vi "Main.vi"() -> ()   [LabVIEW 2015]
uses:
  <vilib>/Analysis/2dsp.llb/2D Complex FFT.vi
  <vilib>/Analysis/NI_AALPro.lvlib
panel:
  in  "Load memory":bool
  out "Trigger mode list":u32[](array[numeric])
  in  "Is record":bool
  in  "Trigger ON/OFF":bool
  in  "Trig send":bool
  in  "live stop":bool
  in  "live start":bool
  out "Error":bool
  out "satus":string
  out "reolsution":cluster{"Width":u32, "Height":u32}
  out "Error_Out":T1
  out "error out":errorcluster
  in  "Stop":bool
  in  "camera parameters":T2={"Setup"={"Shading:"=0, "Partition:"=1, "Shutter:"=0}, "camera"=0, "Head:"=0, "Resolution:"=4, "Frame Rate:"=0, "Camera Option"=FALSE} {"Frame Rate:" items=["50 fps", "60 fps", "125 fps", "250 fps", "500 fps", "1000 fps", "2000 fps", "3000 fps", "3600 fps", "4500 fps", "5000 fps", "6000 fps", "6750 fps", "8000 fps", "10000 fps", "13500 fps", "20000 fps", "30000 fps", "40000 fps", "50000 fps", "60000 fps", "75000 fps", "86400 fps", "100000 fps", "150000 fps", "225000 fps", "360000 fps", "500000 fps"]; "Resolution:" items=["1024 X 1024", "1024 X 896", "1024 X 800", "1024 X 640", "1024 X 512", "896 X 896", "896 X 752", "896 X 640", "896 X 512", "768 X 768", "768 X 640", "768 X 512", "640 X 640", "512 X 512", "512 X 384", "512 X 352", "384 X 288", "320 X 240", "320 X 192", "320 X 160", "320 X 128", "256 X 256", "256 X 128", "256 X 64", "192 X 128", "128 X 128", "128 X 96", "128 X 64", "128 X 32", "128 X 16", "64 X 16"]; "Head:" items=["Head No.0"]; "camera" items=["FASTCAM SA4 model 500K-M1"]; "Setup"."Shutter:" items=["1/50 sec", "1/60 sec", "1/100 sec", "1/200 sec", "1/300 sec", "1/400 sec", "1/500 sec", "1/600 sec", "1/700 sec", "1/800 sec", "1/900 sec", "1/1000 sec", "1/2000 sec", "1/3000 sec", "1/4000 sec", "1/5000 sec", "1/6000 sec", "1/7000 sec", "1/8000 sec", "1/9000 sec", "1/10000 sec", "1/12000 sec", "1/15000 sec", "1/17000 sec", "1/20000 sec", "1/25000 sec", "1/30000 sec", "1/34000 sec", "1/39000 sec", "1/50000 sec", "1/57000 sec", "1/62000 sec", "1/74000 sec", "1/82000 sec", "1/92000 sec", "1/104000 sec", "1/178000 sec", "1/333000 sec", "1/593000 sec", "1/1000000 sec"]; "Setup"."Shading:" items=["Shading"]; "Setup"."Partition:" items=["Partition 1"=1]}
  in  "Tab Control":enum32{"Page 1", "Page 2"}(tab)
  out "Intensity Graph 2":dbl[][](graph)
  out "Intensity Graph":u16[][](graph)
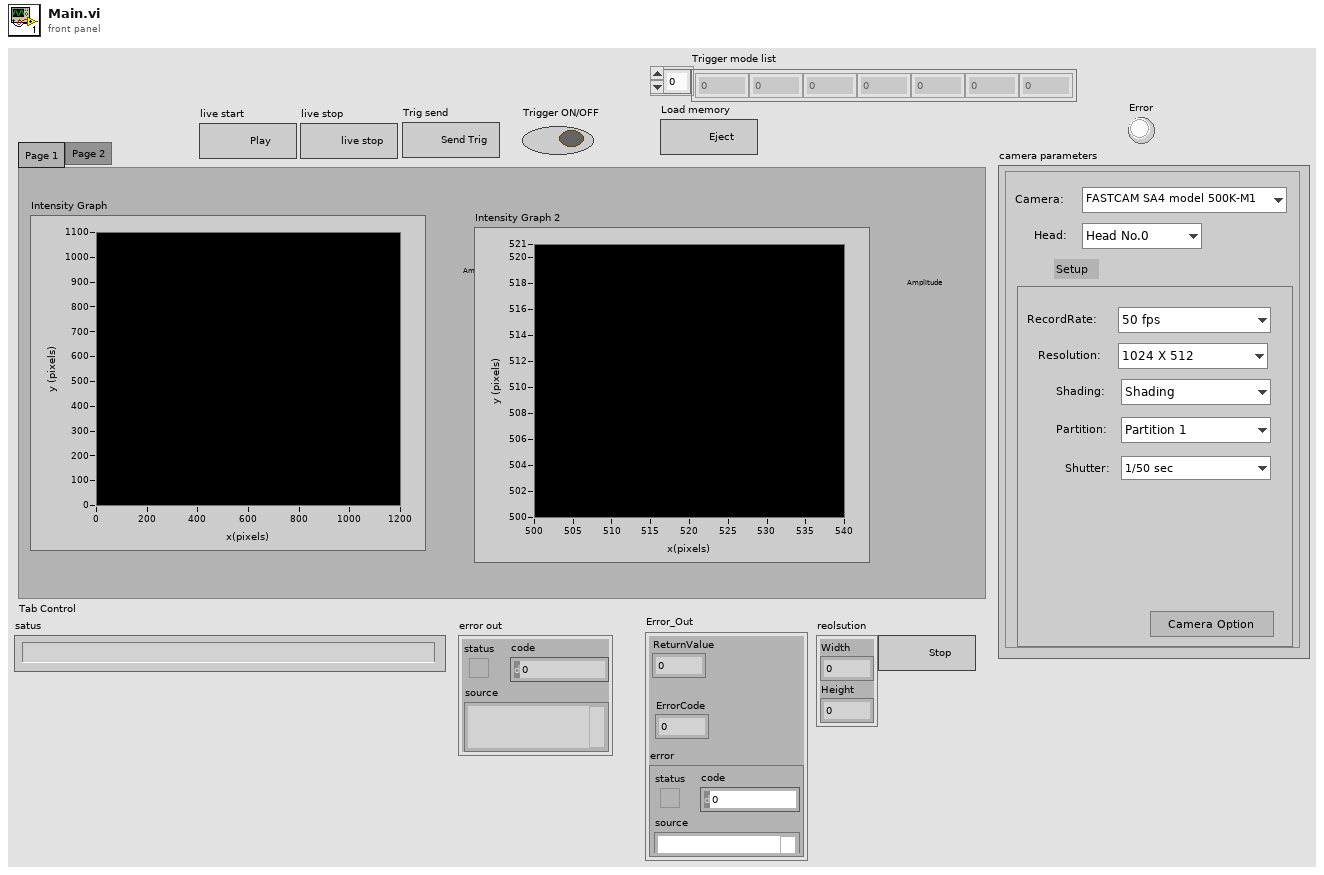
[diagram p1: front panel]
types:
  T1 = cluster{"ReturnValue":u32, "ErrorCode":u32, "error ":errorcluster}
  T2 = cluster{"Setup":cluster{"Shading:":u16, "Partition:":u16, "Shutter:":u16}, "camera":u16, "Head:":u16, "Resolution:":u16, "Frame Rate:":u16, "Camera Option":bool}
  T3 = cluster{"Detect Select BOX":enum32{"Detect Auto", "Detect Normal"}, "Auto_IP":cluster{"IP1":u8, "IP2":u8, "IP3":u8}, "Manual_IP":cluster{"IP1":u8, "IP2":u8, "IP3":u8, "IP4":u8}}
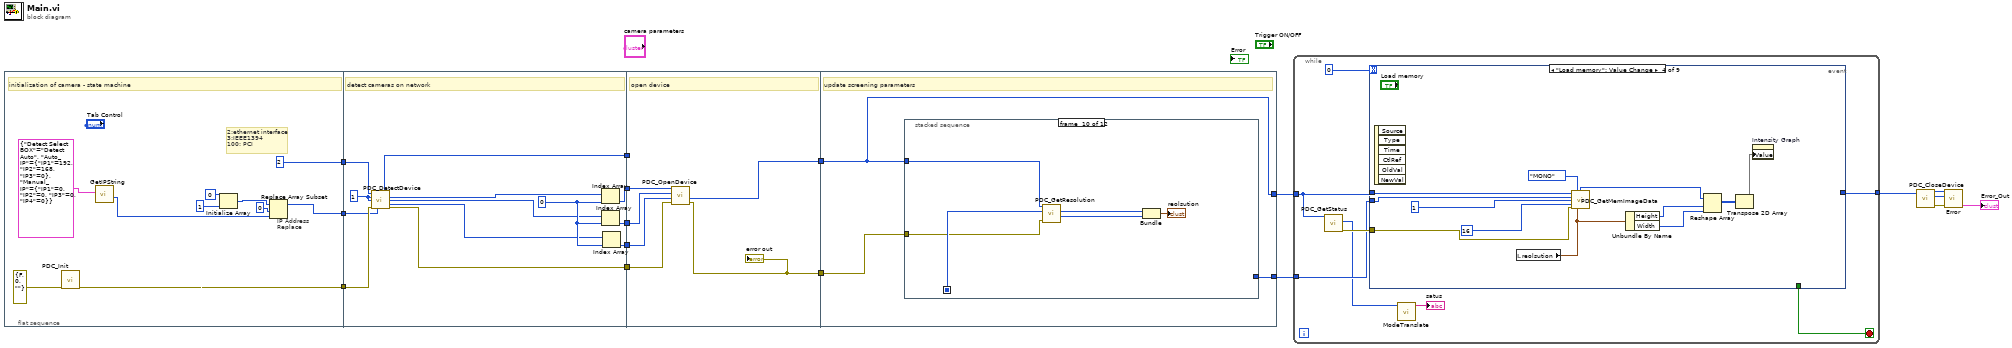
[diagram p0: block diagram]
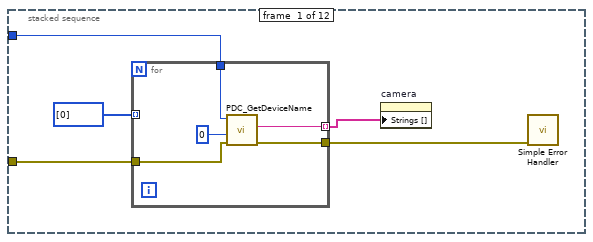
[diagram p2: hidden frame]
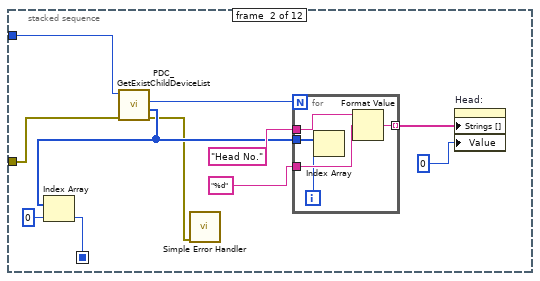
[diagram p3: hidden frame]
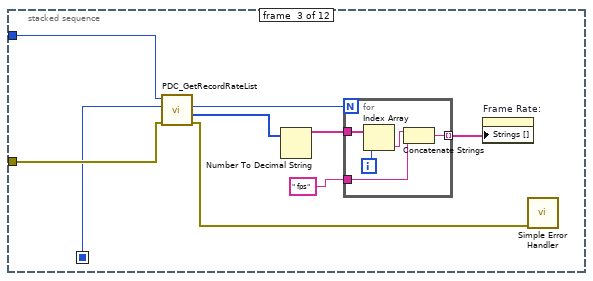
[diagram p4: hidden frame]
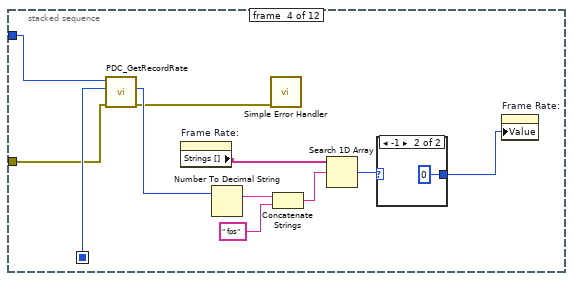
[diagram p5: hidden frame]
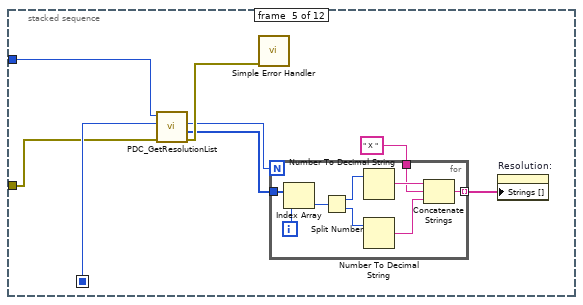
[diagram p7: hidden frame]
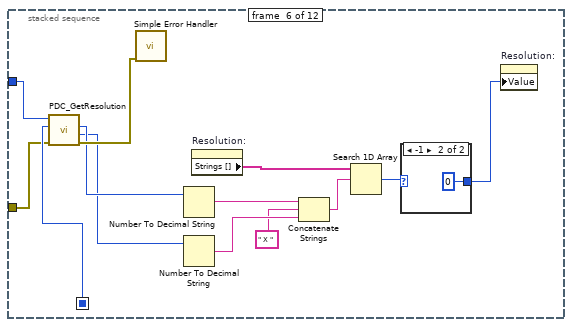
[diagram p8: hidden frame]
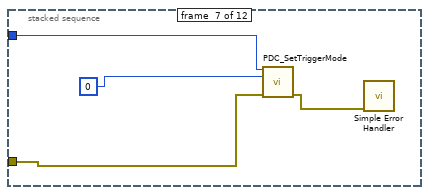
[diagram p10: hidden frame]
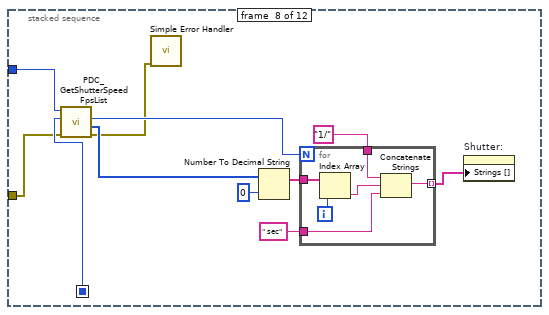
[diagram p11: hidden frame]
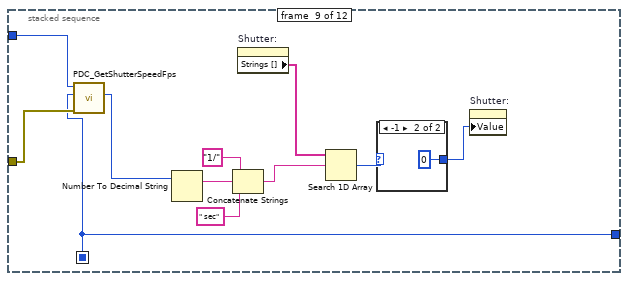
[diagram p12: hidden frame]
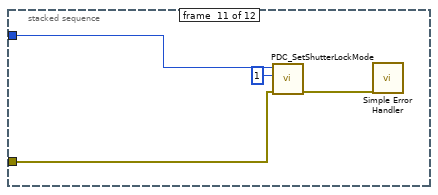
[diagram p14: hidden frame]
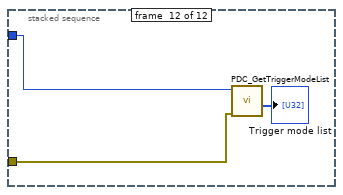
[diagram p15: hidden frame]
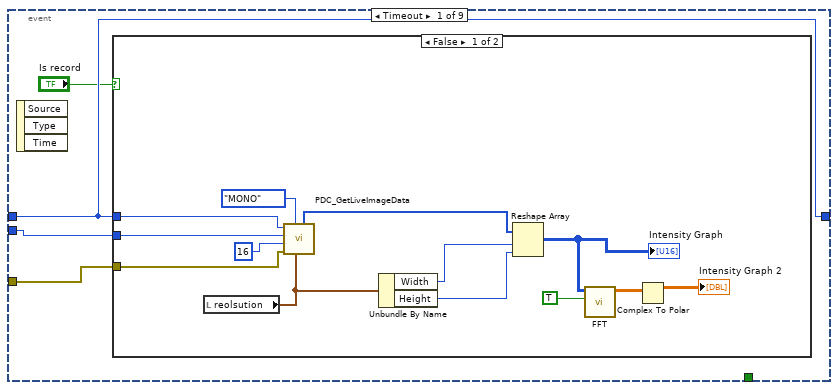
[diagram p16: hidden frame]
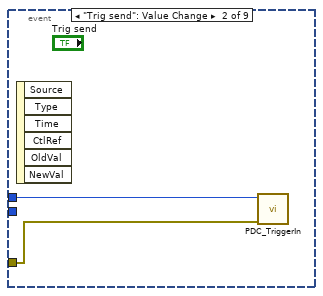
[diagram p18: hidden frame]
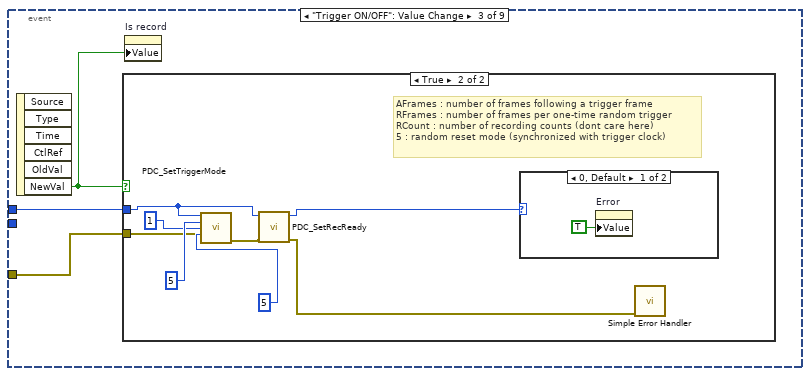
[diagram p19: hidden frame]
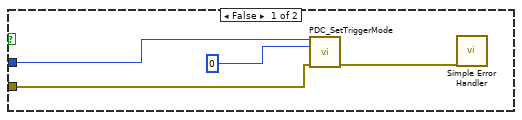
[diagram p20: hidden frame]
diagram:
  n1 = flat-sequence {
    tunnel: [u32 2 ("nInterfaceCode")] -> w17
    tunnel: [w18] -> w16
    tunnel: [w22] -> w15
    tunnel: w17 -> [w38]
    tunnel: w16 -> [w40]
    tunnel: w15 -> [w36]
    tunnel: [w37] -> w14
    tunnel: [w35] -> w13
    tunnel: [w34] -> w12
    tunnel: [w32] -> w11
    tunnel: [w31] -> w2
    tunnel: w14 -> [w43]
    tunnel: w13 -> [w46]
    tunnel: w12 -> [w45]
    tunnel: w11 -> [w44]
    tunnel: [w42] -> w4
    tunnel: [w41] -> w3
    tunnel: w2 -> [_]
    tunnel: [w49] -> w6
    tunnel: w4 -> [w49]
    tunnel: w3 -> [w48]
    tunnel: [w47] -> w1
    frame #0 {
      # "2:ethernet interface\n3:IEEE1394\n100: PCI"
      # "IP Address\nReplace"
      # "initialization of camera - state machine"
      n2 = call "PDC_Init.vi"("error in (no error)"=errorcluster {"status"=FALSE, "code"=0, "source"=""}) -> ("error out"=w18:errorcluster)  [unwired: 10 out]
      n3 = call "GetIPString.vi"("Out_IP Address"=T3 {"Detect Select BOX"=enum."Detect Auto", "Auto_IP"={"IP1"=192, "IP2"=168, "IP3"=0}, "Manual_IP"={"IP1"=0, "IP2"=0, "IP3"=0, "IP4"=0}}) -> ("Net address"=w27:u32)  [unwired: 10 out]
      n4 = Initialize Array "Initialize Array"(u32 0 ("要素"), 1 ("dimension size")) -> (w25:u32[])
      n5 = Replace Array Subset "Replace Array Subset"(array=w25, new element=w27, index=0 ("指標")) -> (w22:u32[])
    }
    frame #1 {
      w33 = 0 ("index")
      w39 = u32 1 ("DetectNum")
      # "detect cameras on network"
      n6 = call "PDC_DetectDevice.vi"("InterfaceCode"=w38, "DetectNum"=w39, "DetectParam"=w39, "error in (no error)"=w40, "DetectNo"=w36) -> ("DeviceNum"=w31:u32, "DeviceCode"=w28:u32[], "TmpDeviceNo"=w30:u32[], "InterfaceCode(out)"=w29:u32[], "error out"=w37:errorcluster)  [unwired: 4 in, 2 out]
      n7 = Index Array(array=w28, index=w33) -> (element=w35:u32)
      n8 = Index Array(array=w30, index=w33) -> (element=w34:u32)
      n9 = Index Array(array=w29, index=w33) -> (element=w32:u32)
    }
    frame #2 {
      # "open device"
      n10 = call "PDC_OpenDevice.vi"("error in (no error)"=w43, "InterfaceCode"=w44, "TmpDeviceNo"=w45, "DeviceCode"=w46) -> ("error out"=w41:errorcluster, "DeviceNo"=w42:u32)  [unwired: 6 out]
      "error out" <- w41
    }
    frame #3 {
      # "update screening parameters"
      n11 = stacked-sequence {
        seq-local: [_ w61 _ _ _ _ _ _ _ _ _ _] -> [_ _ w77 w99 w107 w131 _ w148 w156 w173 _ _]
        tunnel: w49 -> [w54 w70 w84 w100 w108 w132 w138 w149 w166 w174 w178 w181]
        tunnel: w48 -> [w53 w69 w83 w98 w106 w130 w137 w147 w165 w172 w176 w180]
        tunnel: [_ _ _ _ _ _ _ _ w156 _ _ _] -> w47
        frame #0 {
          n12 = for {
            tunnel: w54 -> [w59]
            tunnel: w53 -> [w58]
            tunnel: [w56] -> w51 mode=indexing
            tunnel: u32[] [0] ("nDeviceNoList 2") -> [_] mode=indexing
            tunnel: [w55] -> w50
            n13 = call "PDC_GetDeviceName.vi"("error in (no error)"=w58, "ChildNo"=u32 0, "DeviceNo"=w59) -> ("error out"=w55:errorcluster, "StrName"=w56:string)  [unwired: 1 in, 6 out]
          }
          n14 = property on="camera" class="Ring (strict)"("Strings []"=w51) -> ()  [unwired: 2 in, 2 out]
          n15 = call <vilib>:"Simple Error Handler.vi"("error in (no error)"=w50) -> ()  [unwired: 4 in, 5 out]
        }
        frame #1 {
          n16 = call "PDC_GetExistChildDeviceList.vi"("error in (no error)"=w69, "DeviceNo"=w70) -> ("error out"=w60:errorcluster, "List"=w63:u32[], "Size"=w66:u32)  [unwired: 7 out]
          n17 = Index Array(array=w63, index=0) -> (element=w61:u32)
          n18 = call <vilib>:"Simple Error Handler.vi"("error in (no error)"=w60) -> ()  [unwired: 4 in, 5 out]
          n19 = for {
            N: w66 -> [_]
            tunnel: "Head No." -> [w75]
            tunnel: "%d" -> [w74]
            tunnel: [w73] -> w65 mode=indexing
            tunnel: w63 -> [w71]
            i -> [w72]
            n20 = Index Array(array=w71, index=w72) -> ()  [unwired: 1 out]
            n21 = Format Value(string ("")=w75, format string=w74) -> (output string=w73:string)  [unwired: 1 in]
          }
          n22 = property on="Head:" class="Ring (strict)"("Strings []"=w65, "Value"=u32 0 ("値")) -> ()  [unwired: 2 in, 2 out]
        }
        frame #2 {
          n23 = call "PDC_GetRecordRateList.vi"("error in (no error)"=w83, "ChildNo"=w77, "DeviceNo"=w84) -> ("error out"=w76:errorcluster, "List"=w79:u32[], "Size"=w80:u32)  [unwired: 6 out]
          n24 = Number To Decimal String(number=w79) -> (decimal integer string=w82:string[])  [unwired: 1 out]
          n25 = for {
            N: w80 -> [_]
            tunnel: w82 -> [w86]
            tunnel: [w89] -> w78 mode=indexing
            tunnel: " fps" -> [w88]
            i -> [w87]
            n26 = Index Array(array=w86, index=w87) -> (element=w85:string)
            n27 = Concatenate Strings(w85, w88) -> (w89:string)
          }
          n28 = property on="Frame Rate:" class="Ring (strict)"("Strings []"=w78) -> ()  [unwired: 2 in, 2 out]
          n29 = call <vilib>:"Simple Error Handler.vi"("error in (no error)"=w76) -> ()  [unwired: 4 in, 5 out]
        }
        frame #3 {
          n30 = call "PDC_GetRecordRate.vi"("error in (no error)"=w98, "ChildNo"=w99, "DeviceNo"=w100) -> ("error out"=w90:errorcluster, "Rate"=w91:u32)  [unwired: 7 out]
          n31 = property on="Frame Rate:" class="Ring (strict)"() -> ("Strings []"=w93:string[])  [unwired: 2 in, 2 out]
          n32 = Number To Decimal String(number=w91) -> (decimal integer string=w96:string)  [unwired: 1 out]
          n33 = call <vilib>:"Simple Error Handler.vi"("error in (no error)"=w90) -> ()  [unwired: 4 in, 5 out]
          n34 = Concatenate Strings(w96, " fps") -> (w95:string)
          n35 = Search 1D Array(1D array=w93, element=w95) -> (index of element=w94:i32)  [unwired: 1 out]
          n36 = case shown="-1" w94 {
            selector: w94 -> [w101 _]
            tunnel: [w101 0 ("index of element")] -> w92
            frame Default {
            }
            frame -1 {
            }
          }
          n37 = property on="Frame Rate:" class="Ring (strict)"("Value"=w92) -> ()  [unwired: 2 in, 2 out]
        }
        frame #4 {
          n38 = call "PDC_GetResolutionList.vi"("error in (no error)"=w106, "ChildNo"=w107, "DeviceNo"=w108) -> ("error out"=w105:errorcluster, "List"=w103:u32[], "Size"=w104:u32)  [unwired: 6 out]
          n39 = call <vilib>:"Simple Error Handler.vi"("error in (no error)"=w105) -> ()  [unwired: 4 in, 5 out]
          n40 = for {
            N: w104 -> [_]
            tunnel: " X " -> [w117]
            tunnel: [w116] -> w109 mode=indexing
            tunnel: w103 -> [w112]
            i -> [w115]
            n41 = Index Array(array=w112, index=w115) -> (element=w111:u32)
            n42 = Split Number(x=w111) -> (hi(x)=w114:u16, lo(x)=w113:u16)
            n43 = Number To Decimal String(number=w114) -> (decimal integer string=w119:string)  [unwired: 1 out]
            n44 = Number To Decimal String(number=w113) -> (decimal integer string=w118:string)  [unwired: 1 out]
            n45 = Concatenate Strings(w119, w117, w118) -> (w116:string)
          }
          n46 = property on="Resolution:" class="Ring (strict)"("Strings []"=w109) -> ()  [unwired: 2 in, 2 out]
        }
        frame #5 {
          n47 = call "PDC_GetResolution.vi"("error in (no error)"=w130, "ChildNo"=w131, "DeviceNo"=w132) -> ("error out"=w129:errorcluster, "Height"=w122:u32, "Width"=w123:u32)  [unwired: 6 out]
          n48 = call <vilib>:"Simple Error Handler.vi"("error in (no error)"=w129) -> ()  [unwired: 4 in, 5 out]
          n49 = Number To Decimal String(number=w123) -> (decimal integer string=w126:string)  [unwired: 1 out]
          n50 = Number To Decimal String(number=w122) -> (decimal integer string=w127:string)  [unwired: 1 out]
          n51 = property on="Resolution:" class="Ring (strict)"() -> ("Strings []"=w121:string[])  [unwired: 2 in, 2 out]
          n52 = Concatenate Strings(w126, " X ", w127) -> (w124:string)
          n53 = Search 1D Array(1D array=w121, element=w124) -> (index of element=w128:i32)  [unwired: 1 in]
          n54 = case shown="-1" w128 {
            selector: w128 -> [w133 _]
            tunnel: [w133 0 ("index of element")] -> w120
            frame Default {
            }
            frame -1 {
            }
          }
          n55 = property on="Resolution:" class="Ring (strict)"("Value"=w120) -> ()  [unwired: 2 in, 2 out]
        }
        frame #6 {
          n56 = call "PDC_SetTriggerMode.vi"("DeviceNo"=w138, "Mode"=u32 0 ("nMode"), "error in (no error)"=w137) -> ("error out"=w135:errorcluster)  [unwired: 3 in, 9 out]
          n57 = call <vilib>:"Simple Error Handler.vi"("error in (no error)"=w135) -> ()  [unwired: 4 in, 5 out]
        }
        frame #7 {
          n58 = call "PDC_GetShutterSpeedFpsList.vi"("error in (no error)"=w147, "ChildNo"=w148, "DeviceNo"=w149) -> ("error out"=w139:errorcluster, "List"=w142:u32[], "Size"=w141:u32)  [unwired: 6 out]
          n59 = call <vilib>:"Simple Error Handler.vi"("error in (no error)"=w139) -> ()  [unwired: 4 in, 5 out]
          n60 = Number To Decimal String(number=w142, width (-)=u32 0 ("幅（-）")) -> (decimal integer string=w146:string[])
          n61 = for {
            N: w141 -> [_]
            tunnel: w146 -> [w151]
            tunnel: [w155] -> w140 mode=indexing
            tunnel: "1/" -> [w153]
            tunnel: " sec" -> [w152]
            i -> [w154]
            n62 = Index Array(array=w151, index=w154) -> (element=w150:string)
            n63 = Concatenate Strings(w153, w150, w152) -> (w155:string)
          }
          n64 = property on="Shutter:" class="Ring (strict)"("Strings []"=w140) -> ()  [unwired: 2 in, 2 out]
        }
        frame #8 {
          n65 = call "PDC_GetShutterSpeedFps.vi"("error in (no error)"=w165, "ChildNo"=w156, "DeviceNo"=w166) -> ("Fps"=w157:u32)  [unwired: 8 out]
          n66 = Number To Decimal String(number=w157) -> (decimal integer string=w160:string)  [unwired: 1 out]
          n67 = Concatenate Strings("1/", w160, " sec") -> (w163:string)
          n68 = property on="Shutter:" class="Ring (strict)"() -> ("Strings []"=w158:string[])  [unwired: 2 in, 2 out]
          n69 = Search 1D Array(1D array=w158, element=w163) -> (index of element=w162:i32)  [unwired: 1 out]
          n70 = case shown="-1" w162 {
            selector: w162 -> [w167 _]
            tunnel: [w167 0 ("index of element")] -> w159
            frame Default {
            }
            frame -1 {
            }
          }
          n71 = property on="Shutter:" class="Ring (strict)"("Value"=w159) -> ()  [unwired: 2 in, 2 out]
        }
        frame #9 {
          n72 = call "PDC_GetResolution.vi"("error in (no error)"=w172, "ChildNo"=w173, "DeviceNo"=w174) -> ("Height"=w170:u32, "Width"=w171:u32)  [unwired: 7 out]
          n73 = Bundle("Width"=w171, "Height"=w170) -> (→"reolsution":cluster{"Width":u32, "Height":u32})  [unwired: 1 in]
        }
        frame #10 {
          n74 = call "PDC_SetShutterLockMode.vi"("error in (no error)"=w176, "Mode"=u32 1, "DeviceNo"=w178) -> ("error out"=w175:errorcluster)  [unwired: 6 in, 2 out]
          n75 = call <vilib>:"Simple Error Handler.vi"("error in (no error)"=w175) -> ()  [unwired: 4 in, 5 out]
        }
        frame #11 {
          n76 = call "PDC_GetTriggerModeList.vi"("error in (no error)"=w180, "DeviceNo"=w181) -> ("List"=→"Trigger mode list":u32[])  [unwired: 5 in, 4 out]
        }
      }
    }
  }
  n77 = while {
    tunnel: [w187] -> w7
    tunnel: w6 -> [w188]
    tunnel: w1 -> [w184]
    stop <- w185 stop-if-true
    n78 = call "PDC_GetStatus.vi"("DeviceNo"=w188) -> ("error out"=w186:errorcluster, "Status"=w183:u32)  [unwired: 1 in, 8 out]
    n79 = event shown="[3] \"Load memory\": Value Change" {
      selector: _ -> [_ _ _ _ _ _ _ _ _]
      dyn-events: _ -> [_ _ _ _ _ _ _ _ _]
      timeout: 0 -> [_ _ _ _ _ _ _ _ _]
      tunnel: w188 -> [w192 w208 w211 w236 w241 w244 w247 w268 w269]
      tunnel: [w192 _ _ _ _ _ w247 _ w269] -> w187
      tunnel: w186 -> [w193 w207 w210 w231 w240 w243 w255 w266 _]
      tunnel: [_ _ _ _ _ _ _ _ TRUE] -> w185
      tunnel: w184 -> [w191 _ _ w234 _ _ w246 w267 _]
      event Timeout {
        n80 = event-data() -> ()  [unwired: 1 in, 3 out]
        n81 = case shown="False" "Is record" {
          tunnel: w193 -> [w204 _]
          tunnel: w192 -> [w199 _]
          tunnel: w191 -> [w198 _]
          frame False {
            n82 = local read "reolsution"() -> (w202:cluster{"Width":u32, "Height":u32})
            n83 = call "PDC_GetLiveImageData.vi"("Resolution"=w202, "ColorType"=enum16{"MONO", "COLOR"}."MONO", "error in (no error)"=w204, "BitDepth"=u32 16, "ChildNo"=w198, "DeviceNo"=w199) -> ("Data(16Bit)"=w203:u16[])  [unwired: 5 out]
            n84 = Unbundle By Name(w202) -> ("Width"=w201:u32, "Height"=w200:u32)
            n85 = Reshape Array(w203, w201, w200) -> (w197:u16[][])
            "Intensity Graph" <- w197
            n86 = call-poly <vilib>:"FFT.vi"("shift?"=TRUE, "X"=w197) -> ("FFT {X}"=w196:cdb[][])  [unwired: 8 in, 1 out]
            n87 = Complex To Polar(r * e^(i*theta)=w196) -> (r=→"Intensity Graph 2":dbl[][])  [unwired: 1 out]
          }
          frame True {
          }
        }
      }
      event "Trig send": Value Change {
        n88 = event-data() -> ()  [unwired: 1 in, 6 out]
        n89 = call "PDC_TriggerIn.vi"("error in (no error)"=w207, "DeviceNo"=w208) -> ()  [unwired: 7 in, 3 out]
      }
      event "Trigger ON/OFF": Value Change {
        n90 = event-data() -> ("NewVal"=w209:bool)  [unwired: 1 in, 5 out]
        n91 = case shown="True" w209 {
          tunnel: w211 -> [w214 w216]
          tunnel: w210 -> [w212 w220]
          frame False {
            n92 = call "PDC_SetTriggerMode.vi"("DeviceNo"=w214, "Mode"=u32 0, "error in (no error)"=w212) -> ("error out"=w215:errorcluster)  [unwired: 10 in, 2 out]
            n93 = call <vilib>:"Simple Error Handler.vi"("error in (no error)"=w215) -> ()  [unwired: 4 in, 5 out]
          }
          frame True {
            # "AFrames : number of frames following a trigger frame\nRFrames : number of frames per one-time random trigger\nRCount : number of recording counts (dont care here)\n5 : random reset mode (synchronized with trigger clock)"
            n94 = call "PDC_SetTriggerMode.vi"("DeviceNo"=w216, "Mode"=u32 5, "AFrames"=u32 1, "RFrames"=u32 5, "error in (no error)"=w220) -> ("error out"=w219:errorcluster)  [unwired: 8 in, 2 out]
            n95 = call "PDC_SetRecReady.vi"("error in (no error)"=w219, "DeviceNo"=w216) -> ("error out"=w218:errorcluster, "ReturnValue"=w217:u32)  [unwired: 7 in, 1 out]
            n96 = case shown="0, Default" w217 {
              frame 0, Default {
                n97 = property on="Error" class="Bool (strict)"("Value"=TRUE ("Error")) -> ()  [unwired: 2 in, 2 out]
              }
              frame 1 {
              }
            }
            n98 = call <vilib>:"Simple Error Handler.vi"("error in (no error)"=w218) -> ()  [unwired: 4 in, 5 out]
          }
        }
        n99 = property on="Is record" class="Bool (strict)"("Value"=w209) -> ()  [unwired: 2 in, 2 out]
      }
      event "Load memory": Value Change {
        n100 = event-data() -> ()  [unwired: 1 in, 6 out]
        n101 = local read "reolsution"() -> (w230:cluster{"Width":u32, "Height":u32})
        n102 = call "PDC_GetMemImageData.vi"("DeviceNo"=w236, "ColorType"=enum16{"MONO", "COLOR"}."MONO", "ChildNo"=w234, "FrameNo"=1, "BitDepth"=u32 16, "error in (no error)"=w231, "Resolution"=w230) -> ("Data(16Bit)"=w227:u16[])  [unwired: 4 in, 4 out]
        n103 = Unbundle By Name(w230) -> ("Height"=w229:u32, "Width"=w228:u32)
        n104 = Reshape Array(w227, w229, w228) -> (w226:u16[][])
        n105 = Transpose 2D Array(2D array=w226) -> (transposed array=w225:u16[][])
        n106 = property on="Intensity Graph" class="IntGraph (strict)"("Value"=w225) -> ()  [unwired: 2 in, 2 out]
      }
      event "live stop": Value Change {
        n107 = event-data() -> ()  [unwired: 1 in, 6 out]
        n108 = call "PDC_SetStatus.vi"("error in (no error)"=w240, "Mode"=u32 1, "DeviceNo"=w241) -> ("error out"=w239:errorcluster)  [unwired: 8 out]
        n109 = call <vilib>:"Simple Error Handler.vi"("error in (no error)"=w239) -> ()  [unwired: 4 in, 5 out]
        n110 = property on="Is record" class="Bool (strict)"("Value"=TRUE ("Is live")) -> ()  [unwired: 2 in, 2 out]
      }
      event "live start": Value Change {
        n111 = event-data() -> ()  [unwired: 1 in, 6 out]
        n112 = call "PDC_SetStatus.vi"("error in (no error)"=w243, "Mode"=u32 0, "DeviceNo"=w244) -> ()  [unwired: 9 out]
        n113 = property on="Is record" class="Bool (strict)"("Value"=FALSE ("Is live")) -> ()  [unwired: 2 in, 2 out]
      }
      event "camera parameters.Frame Rate:": Value Change {
        n114 = event-data() -> ()  [unwired: 1 in, 6 out]
        n115 = property on="Frame Rate:" class="Ring (strict)"() -> ("Strings []"=w250:string[], "Value"=w249:u16)  [unwired: 2 in, 2 out]
        n116 = Index Array(array=w250, index=w249) -> (element=w254:string)
        n117 = Match Pattern(string=w254, regular expression=" fps") -> (before substring=w252:string)  [unwired: 4 out]
        n118 = Decimal String To Number(string=w252, default (0L)=u32 0 ("デフォルト (0 I32)")) -> (number=w248:u32)  [unwired: 2 out]
        n119 = call "PDC_SetRecordRate.vi"("error in (no error)"=w255, "Rate"=w248, "ChildNo"=w246, "DeviceNo"=w247) -> ("error out"=w256:errorcluster)  [unwired: 7 out]
        n120 = call <vilib>:"Simple Error Handler.vi"("error in (no error)"=w256) -> ()  [unwired: 4 in, 5 out]
      }
      event "camera parameters.Setup.Shutter:": Value Change {
        n121 = event-data() -> ()  [unwired: 1 in, 6 out]
        n122 = property on="Shutter:" class="Ring (strict)"() -> ("Strings []"=w258:string[], "Value"=w257:u16)  [unwired: 2 in, 2 out]
        n123 = Index Array(array=w258, index=w257) -> (element=w265:string)
        n124 = Match Pattern(string=w265, regular expression=" sec") -> (before substring=w262:string)  [unwired: 4 out]
        n125 = Match Pattern(string=w262, regular expression="1/") -> (after substring=w260:string)  [unwired: 4 out]
        n126 = Decimal String To Number(string=w260, default (0L)=u32 0 ("デフォルト (0 I32)")) -> (number=w259:u32)  [unwired: 2 out]
        n127 = call "PDC_SetShutterSpeedFps.vi"("error in (no error)"=w266, "Fps"=w259, "ChildNo"=w267, "DeviceNo"=w268) -> ()  [unwired: 8 out]
      }
      event "Stop": Value Change {
        n128 = event-data() -> ()  [unwired: 1 in, 6 out]
      }
    }
    n129 = call "ModeTranslate.vi"("Status 2"=w183) -> ("String"=→"satus":string)  [unwired: 10 in]
  }
  n130 = call "PDC_CloseDevice.vi"("DeviceNo"=w7) -> ("error out"=w8:errorcluster, "ErrorCode"=w9:u32, "ReturnValue"=w10:u32)  [unwired: 4 in, 4 out]
  n131 = call "Error.vi"("error in (no error)"=w8, "ErrorCode"=w9, "ReturnValue"=w10) -> ("Error_Out"=→"Error_Out":T1)  [unwired: 8 out]
